vi "toml_api_type_cast.vi"(7 "action":enum8{"get", "set"}(ring), 8 "error in (no error)":errorcluster, 10 "item":T2, 11 "sections in":T1(array[cluster])) -> (0 "error out":errorcluster, 1 "exists?":bool, 2 "value":variant, 3 "sections out":T1(array[cluster]))   [LabVIEW 2017]
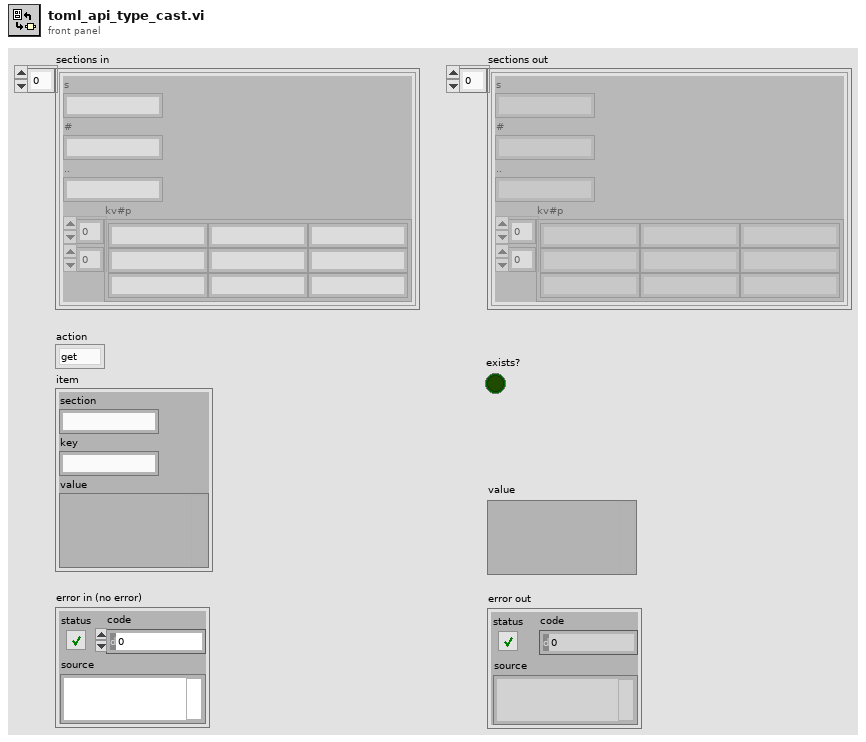
[diagram p1: front panel]
types:
  T1 = cluster{"s":string, "#":string, "..":string, "kv#p":string[][]}[]
  T2 = cluster{"section":string, "key":string, "value":variant}
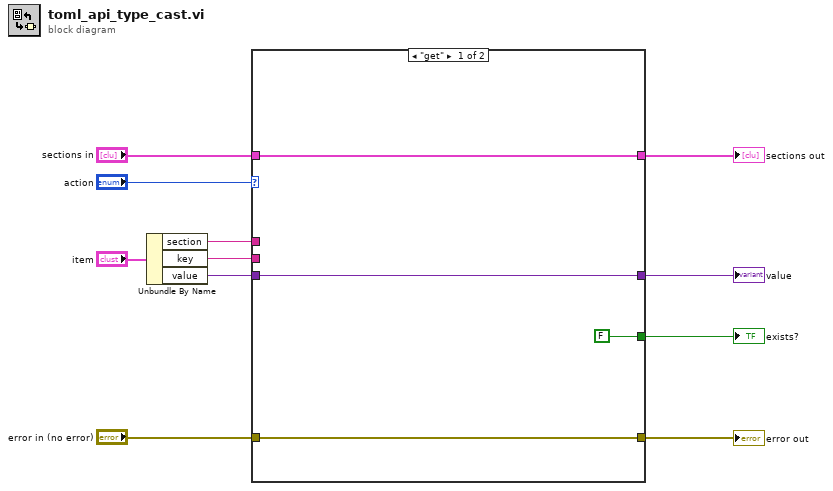
[diagram p0: block diagram]
diagram:
  n1 = Unbundle By Name("item") -> ("section"=w7:string, "key"=w6:string, "value"=w5:variant)
  n2 = case shown="\"get\"" "action" {
    tunnel: [w15 w18] -> w1
    tunnel: "sections in" -> [w15 w18]
    tunnel: [w14 w17] -> w9
    tunnel: "error in (no error)" -> [w14 w17]
    tunnel: w7 -> [_ _]
    tunnel: w6 -> [_ _]
    tunnel: w5 -> [w13 w16]
    tunnel: [w13 w16] -> w4
    tunnel: [FALSE ("exists?") _] -> w3
    frame "get" {
    }
    frame "set" {
    }
  }
  "error out" <- w9
  "value" <- w4
  "exists?" <- w3
  "sections out" <- w1
